vi "gentec-SOLO-PE.Offsetter.vi"(0 "Value":dbl format="%.12f") -> (1 "Value":u32, 2 "Scale":T1 items=["Auto", "1 pJ", "3 pJ", "10 pJ", "30 pJ", "100 pJ", "300 pJ", "1 nJ", "3 nJ", "10 nJ", "30 nJ", "100 nJ", "300 nJ", "1 uJ", "3 uJ", "10 uJ", "30 uJ", "100 uJ", "300 uJ", "1 mJ", "3 mJ", "10 mJ", "30 mJ", "100 mJ", "300 mJ", "1 J", "3 J", "10 J", "30 J", "100 J", "300 J", "1 kJ", "3 kJ", "10 kJ", "30 kJ", "100 kJ", "300 kJ", "1 MJ", "3 MJ", "10 MJ", "30 MJ", "100 MJ", "300 MJ"])   [LabVIEW 2014, in "gentec-SOLO-PE - Driver.lvlib"]
uses:
  gentec-SOLO-PE - Driver.lvlib
  Type Defs/gentec-SOLO-PE.Scale.ctl
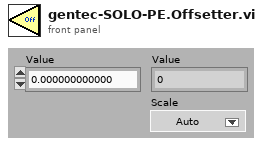
[diagram p1: front panel]
types:
  T1 = typedef "gentec-SOLO-PE - Driver.lvlib/gentec-SOLO-PE.Scale.ctl" = u32
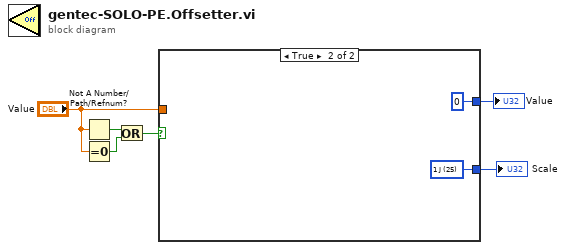
[diagram p0: block diagram]
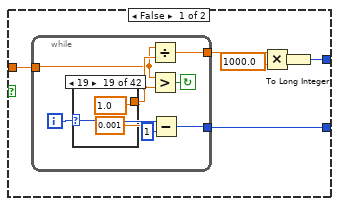
[diagram p2: hidden frame]
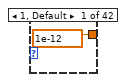
[diagram p3: hidden frame]
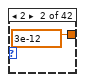
[diagram p4: hidden frame]
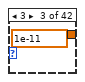
[diagram p5: hidden frame]
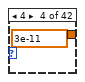
[diagram p6: hidden frame]
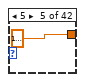
[diagram p7: hidden frame]
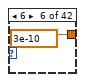
[diagram p8: hidden frame]
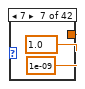
[diagram p9: hidden frame]
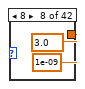
[diagram p10: hidden frame]
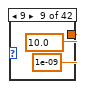
[diagram p11: hidden frame]
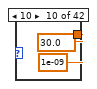
[diagram p12: hidden frame]
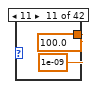
[diagram p13: hidden frame]
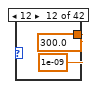
[diagram p14: hidden frame]
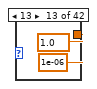
[diagram p15: hidden frame]
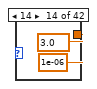
[diagram p16: hidden frame]
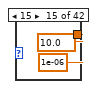
[diagram p17: hidden frame]
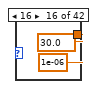
[diagram p18: hidden frame]
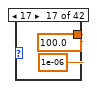
[diagram p19: hidden frame]
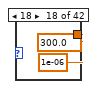
[diagram p20: hidden frame]
diagram:
  n1 = Not A Number/Path/Refnum?(number/path/refnum="Value") -> (NaN/Path/Refnum?=w3:bool)
  n2 = Equal To 0?(x="Value") -> (x = 0?=w2:bool)
  n3 = Or(x=w3, y=w2) -> (x .or. y?=w1:bool)
  n4 = case shown="True" w1 {
    tunnel: [w12 0] -> w6
    tunnel: [w11 w134] -> w5
    tunnel: "Value" -> [w7 _]
    frame False {
      n5 = while {
        tunnel: w7 -> [w17]
        tunnel: [w14] -> w11
        tunnel: [w16] -> w9
        i -> [w15]
        stop <- w19 continue-if-true
        n6 = case shown="19" w15 {
          tunnel: [1e-12 3e-12 1e-11 3e-11 1e-10 3e-10 w28 w31 w34 w37 w40 w43 w46 w49 w52 w55 w58 w61 w64 w67 w70 w73 w76 w79 w82 w85 w86 w89 w94 w97 w100 w103 w106 w109 w112 w115 w118 w121 w124 w127 w130 w133] -> w18
          frame 1, Default {
          }
          frame 2 {
          }
          frame 3 {
          }
          frame 4 {
          }
          frame 5 {
          }
          frame 6 {
          }
          frame 7 {
            n7 = Multiply(x=1.0, y=1e-09) -> (x*y=w28:dbl)
          }
          frame 8 {
            n8 = Multiply(x=3.0, y=1e-09) -> (x*y=w31:dbl)
          }
          frame 9 {
            n9 = Multiply(x=10.0, y=1e-09) -> (x*y=w34:dbl)
          }
          frame 10 {
            n10 = Multiply(x=30.0, y=1e-09) -> (x*y=w37:dbl)
          }
          frame 11 {
            n11 = Multiply(x=100.0, y=1e-09) -> (x*y=w40:dbl)
          }
          frame 12 {
            n12 = Multiply(x=300.0, y=1e-09) -> (x*y=w43:dbl)
          }
          frame 13 {
            n13 = Multiply(x=1.0, y=1e-06) -> (x*y=w46:dbl)
          }
          frame 14 {
            n14 = Multiply(x=3.0, y=1e-06) -> (x*y=w49:dbl)
          }
          frame 15 {
            n15 = Multiply(x=10.0, y=1e-06) -> (x*y=w52:dbl)
          }
          frame 16 {
            n16 = Multiply(x=30.0, y=1e-06) -> (x*y=w55:dbl)
          }
          frame 17 {
            n17 = Multiply(x=100.0, y=1e-06) -> (x*y=w58:dbl)
          }
          frame 18 {
            n18 = Multiply(x=300.0, y=1e-06) -> (x*y=w61:dbl)
          }
          frame 19 {
            n19 = Multiply(x=1.0, y=0.001) -> (x*y=w64:dbl)
          }
          frame 20 {
            n20 = Multiply(x=3.0, y=0.001) -> (x*y=w67:dbl)
          }
          frame 21 {
            n21 = Multiply(x=10.0, y=0.001) -> (x*y=w70:dbl)
          }
          frame 22 {
            n22 = Multiply(x=30.0, y=0.001) -> (x*y=w73:dbl)
          }
          frame 23 {
            n23 = Multiply(x=100.0, y=0.001) -> (x*y=w76:dbl)
          }
          frame 24 {
            n24 = Multiply(x=300.0, y=0.001) -> (x*y=w79:dbl)
          }
          frame 25 {
            n25 = Multiply(x=1.0, y=1.0) -> (x*y=w82:dbl)
          }
          frame 26 {
            n26 = Multiply(x=3.0, y=1.0) -> (x*y=w85:dbl)
          }
          frame 28 {
            n27 = Multiply(x=30.0, y=1.0) -> (x*y=w86:dbl)
          }
          frame 29 {
            n28 = Multiply(x=100.0, y=1.0) -> (x*y=w89:dbl)
          }
          frame 27 {
            n29 = Multiply(x=10.0, y=1.0) -> (x*y=w94:dbl)
          }
          frame 30 {
            n30 = Multiply(x=300.0, y=1.0) -> (x*y=w97:dbl)
          }
          frame 31 {
            n31 = Multiply(x=1.0, y=1000.0) -> (x*y=w100:dbl)
          }
          frame 32 {
            n32 = Multiply(x=3.0, y=1000.0) -> (x*y=w103:dbl)
          }
          frame 33 {
            n33 = Multiply(x=10.0, y=1000.0) -> (x*y=w106:dbl)
          }
          frame 34 {
            n34 = Multiply(x=30.0, y=1000.0) -> (x*y=w109:dbl)
          }
          frame 35 {
            n35 = Multiply(x=100.0, y=1000.0) -> (x*y=w112:dbl)
          }
          frame 36 {
            n36 = Multiply(x=300.0, y=1000.0) -> (x*y=w115:dbl)
          }
          frame 37 {
            n37 = Multiply(x=1.0, y=1000000.0) -> (x*y=w118:dbl)
          }
          frame 38 {
            n38 = Multiply(x=3.0, y=1000000.0) -> (x*y=w121:dbl)
          }
          frame 39 {
            n39 = Multiply(x=10.0, y=1000000.0) -> (x*y=w124:dbl)
          }
          frame 40 {
            n40 = Multiply(x=30.0, y=1000000.0) -> (x*y=w127:dbl)
          }
          frame 41 {
            n41 = Multiply(x=100.0, y=1000000.0) -> (x*y=w130:dbl)
          }
          frame 42 {
            n42 = Multiply(x=300.0, y=1000000.0) -> (x*y=w133:dbl)
          }
        }
        n43 = Divide(x=w17, y=w18) -> (x/y=w16:dbl)
        n44 = Greater?(x=w17, y=w18) -> (0:w19:bool)
        n45 = Subtract(x=w15, y=1) -> (x-y=w14:i32)
      }
      n46 = Multiply(x=w9, y=1000.0) -> (x*y=w10:dbl)
      n47 = To Long Integer(number=w10) -> (32bit integer=w12:i32)
    }
    frame True {
      w134 = T1 25 items=["Auto", "1 pJ", "3 pJ", "10 pJ", "30 pJ", "100 pJ", "300 pJ", "1 nJ", "3 nJ", "10 nJ", "30 nJ", "100 nJ", "300 nJ", "1 uJ", "3 uJ", "10 uJ", "30 uJ", "100 uJ", "300 uJ", "1 mJ", "3 mJ", "10 mJ", "30 mJ", "100 mJ", "300 mJ", "1 J", "3 J", "10 J", "30 J", "100 J", "300 J", "1 kJ", "3 kJ", "10 kJ", "30 kJ", "100 kJ", "300 kJ", "1 MJ", "3 MJ", "10 MJ", "30 MJ", "100 MJ", "300 MJ"] ("Scale")
    }
  }
  "Value" <- w6
  "Scale" <- w5
